vi "GyroscopeClose.vi"(8 "error in":errorcluster, 11 "Device In":u64) -> (0 "error out":errorcluster)   [LabVIEW 2020, in "Phidget Gyroscope.lvlib"]
doc: "${Gyroscope:CloseHeader}"
uses:
  <instrlib>/Phidgets/Phidget Gyroscope/Phidget Gyroscope.lvlib
  <instrlib>/Phidgets/Phidget Common/Phidget Common.lvlib
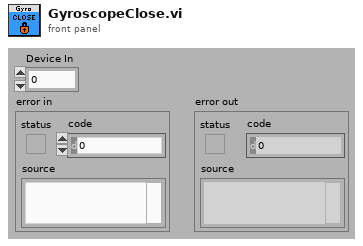
[diagram p1: front panel]
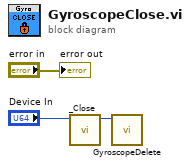
[diagram p0: block diagram]
diagram:
  n1 = call <instrlib>:"_Close.vi"("Device In"="Device In") -> ("Device Out"=w1:u64)  [unwired: 9 in, 1 out]
  n2 = call <instrlib>:"GyroscopeDelete.vi"("Device In"=w1) -> ()  [unwired: 10 in, 1 out]
  "error out" <- "error in"
